vi "Calibrate and Load.vi"(8 "Calibration Cluster":T1, 9 "Always Calibrate":bool, 10 "Do Not Calibrate":bool, 11 "IO Cluster In":T2={"Error"={"status"=FALSE, "code"=0, "source"=""}, "Encoder Calibration Values"=[22, 216], "Update Calibration"=FALSE, "JPEG Resolutions"=3, "Raw Resolutions"=1, "Image Mode"=enum."RAW Gray Scale", "FPGA Ref"=refnum} {"JPEG Resolutions" items=["160x128"=3, "320x240"=5, "640x480"=7]; "Raw Resolutions" items=["80x60"=1, "160x120"=3, "128x128"=9, "128x96"=11]}) -> (0 "Exit Loop":bool, 2 "State Out":T3, 3 "IO Cluster Out":T2={"Error"={"status"=FALSE, "code"=0, "source"=""}, "Encoder Calibration Values"=[22, 216], "Update Calibration"=FALSE, "JPEG Resolutions"=3, "Raw Resolutions"=1, "Image Mode"=enum."RAW Gray Scale", "FPGA Ref"=refnum} {"JPEG Resolutions" items=["160x128"=3, "320x240"=5, "640x480"=7]; "Raw Resolutions" items=["80x60"=1, "160x120"=3, "128x128"=9, "128x96"=11]})   [LabVIEW 2019]
uses:
  Operation States.ctl
  QNET MS IO Cluster.ctl
  <vilib>/Utility/error.llb/Error Cluster From Error Code.vi
  <vilib>/rvi/errors/niLvFpgaAdjustHostInterfaceError.vi
  <vilib>/rvi/interface/nirviReadWriteControl/nirviReadWriteControl.xnode
  NiFpgaLv.dll
  <vilib>/rvi/interface/Simulation/niFpgaSimulationCallBeginRW.vi
panel:
  out "Close Enough?":bool
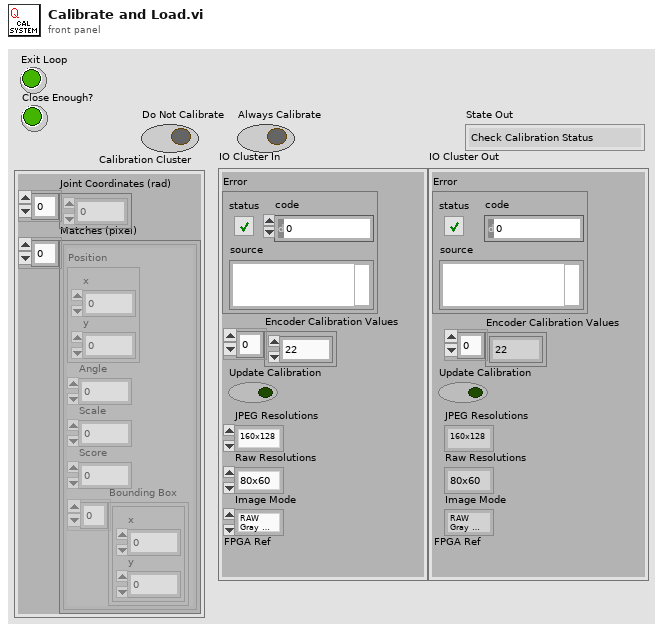
[diagram p1: front panel]
types:
  T1 = cluster{"Joint Coordinates (rad)":dbl[], "Matches (pixel)":cluster{"Position":cluster{"x":sgl, "y":sgl}, "Angle":sgl, "Scale":sgl, "Score":sgl, "Bounding Box":cluster{"x":sgl, "y":sgl}[]}[]}
  T2 = typedef "QNET MS IO Cluster.ctl" = cluster{"Error":errorcluster, "Encoder Calibration Values":i32[], "Update Calibration":bool, "JPEG Resolutions":u16, "Raw Resolutions":u16, "Image Mode":enum16{"RAW RGB", "RAW Gray Scale", "JPEG"}, "FPGA Ref":refnum<k20>}
  T3 = typedef "Operation States.ctl" = enum16{"Check Calibration Status", "Move to Hard Stops", "Calibrate on Symbol", "Calibration Done"}
  T4 = cluster{"Position":cluster{"x":sgl, "y":sgl}, "Angle":sgl, "Scale":sgl, "Score":sgl, "Bounding Box":cluster{"x":sgl, "y":sgl}[]}[]
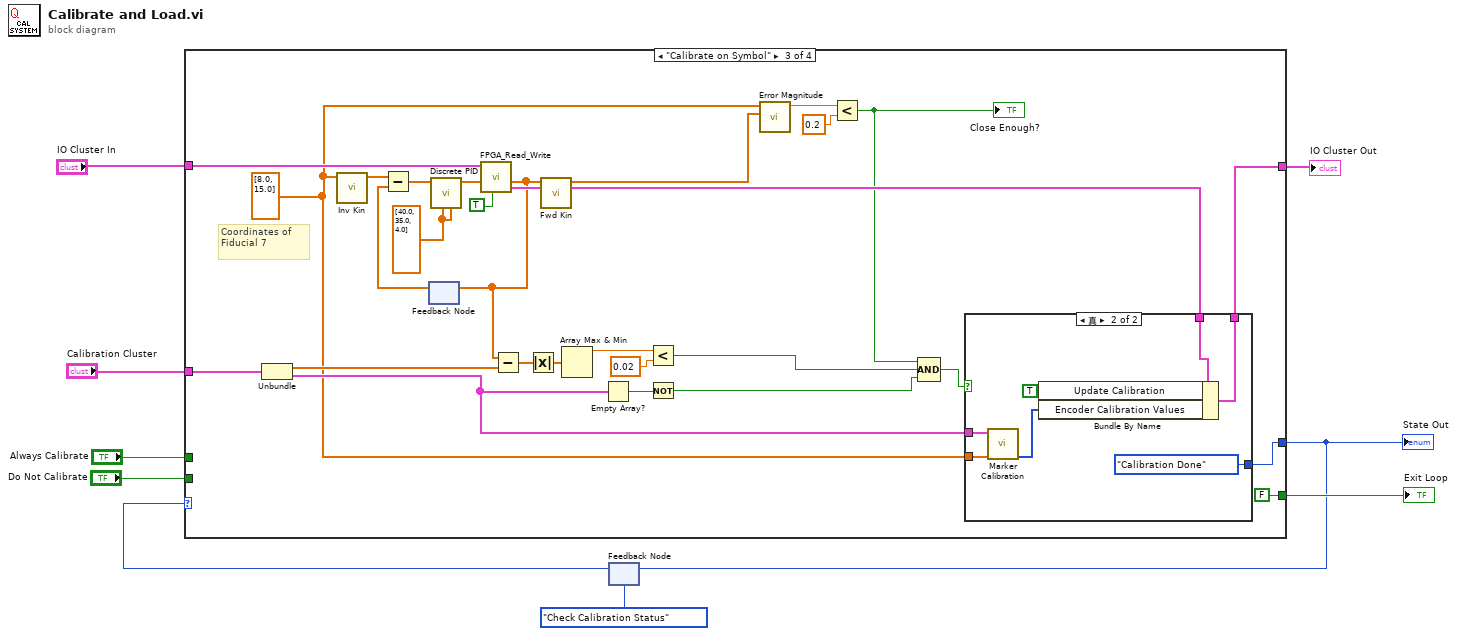
[diagram p0: block diagram]
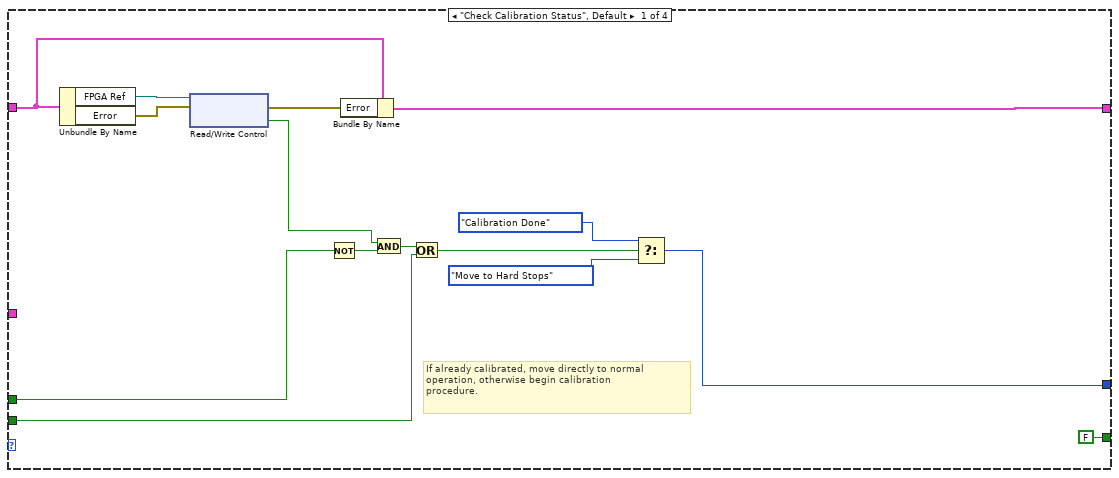
[diagram p2: hidden frame]
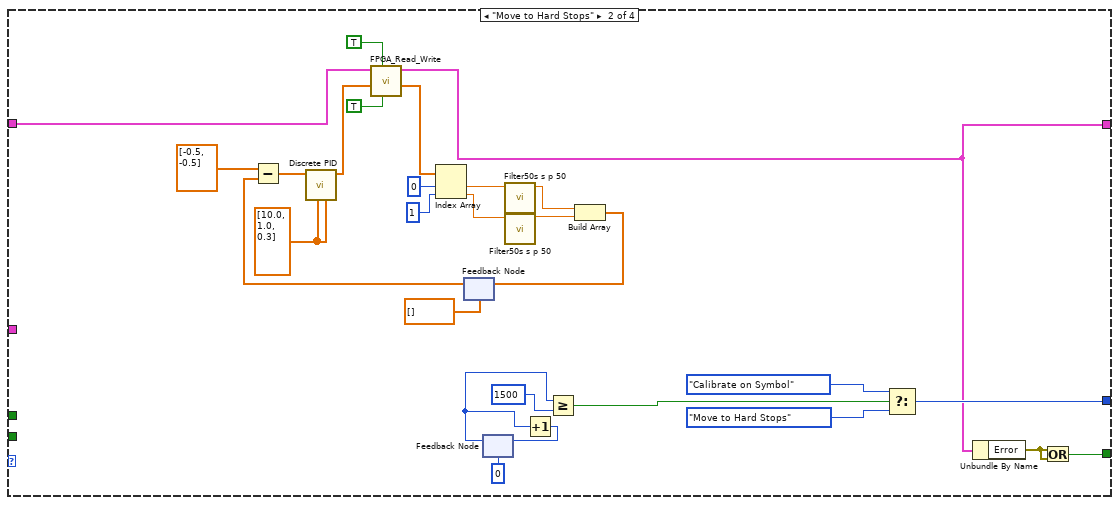
[diagram p3: hidden frame]
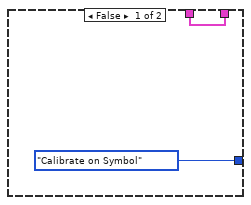
[diagram p4: hidden frame]
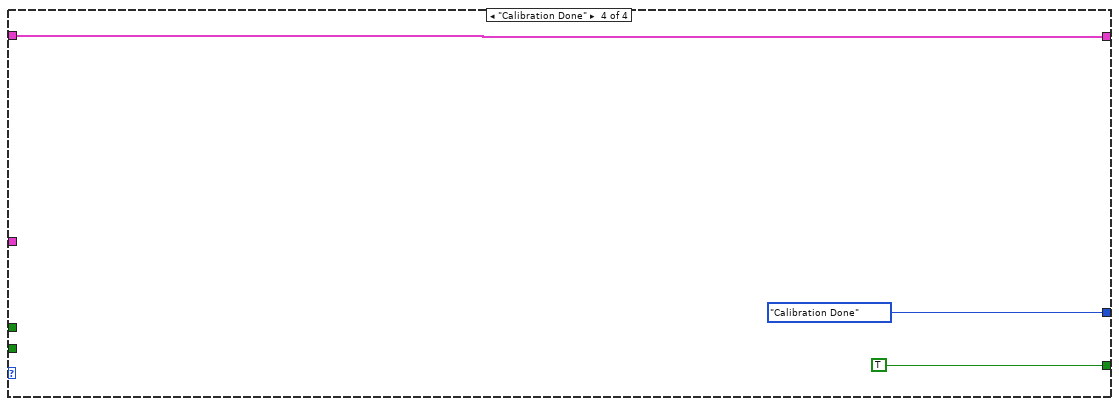
[diagram p5: hidden frame]
diagram:
  n1 = feedback #1(Operation_States."Check Calibration Status") -> (w6:T3)
  n2 = case shown="\"Calibrate on Symbol\"" w6 {
    tunnel: "IO Cluster In" -> [w21 w31 w80 w91]
    tunnel: [FALSE w46 FALSE TRUE] -> w9
    tunnel: [w11 w28 w73 w91] -> w3
    tunnel: [w19 w50 w65 Operation_States."Calibration Done"] -> w5
    tunnel: "Always Calibrate" -> [w16 _ _ _]
    tunnel: "Do Not Calibrate" -> [w13 _ _ _]
    tunnel: "Calibration Cluster" -> [_ _ w68 _]
    frame "Check Calibration Status", Default {
      # "If already calibrated, move directly to normal\noperation, otherwise begin calibration\nprocedure."
      n3 = Unbundle By Name(w21) -> ("FPGA Ref"=w23:refnum<k20>, "Error"=w22:errorcluster)
      n4 = xnode "Read/Write Control"("FPGA VI引用输入"=w23, "错误输入"=w22) -> ("错误输出"=w24:errorcluster, "Calibrated"=w15:bool)  [unwired: 1 out]
      n5 = Not(x=w16) -> (.not. x?=w17:bool)
      n6 = Bundle By Name(cluster=w21, "Error"=w24) -> (w11:T2)
      n7 = And(x=w15, y=w17) -> (x .and. y?=w14:bool)
      n8 = Or(x=w14, y=w13) -> (x .or. y?=w12:bool)
      n9 = Select(t=Operation_States."Calibration Done", s=w12, f=Operation_States."Move to Hard Stops") -> (s? t:f=w19:T3)
    }
    frame "Move to Hard Stops" {
      w35 = dbl[] [10.0, 1.0, 0.3] ("Gains Motor 1")
      n10 = feedback #2(dbl[] []) -> (w38:dbl[])
      n11 = Subtract(x=dbl[] [-0.5, -0.5], y=w38) -> (x-y=w36:dbl[])
      n12 = call "Discrete PID.vi"("Gains Motor 1"=w35, "Gains Motor 0"=w35, "Error Array"=w36) -> ("Voltage"=w25:dbl[])  [unwired: 8 in]
      n13 = call "FPGA_Read_Write.vi"("Motors enabled?"=TRUE, "Reset Encoders?"=TRUE, "Commands"=w25, "IO Cluster In"=w31) -> ("Joint Coordinates (rad)"=w29:dbl[], "IO Cluster Out"=w28:T2)  [unwired: 4 in, 2 out]
      n14 = Index Array(array=w29, index #1=0 ("index"), index #2=1 ("index 2")) -> (element #1=w43:dbl, element #2=w42:dbl)
      n15 = feedback #3(0 ("x")) -> (w32:i32)
      n16 = call "Filter50s s p 50.vi"("u"=w43) -> ("y"=w41:dbl)  [unwired: 10 in]
      n17 = call "Filter50s s p 50.vi"("u"=w42) -> ("y"=w40:dbl)  [unwired: 10 in]
      n18 = Increment(x=w32) -> (x+1=w51:i32)
      n19 = feedback-in #3(w51) -> ()
      n20 = Greater Or Equal?(x=w32, y=1500 ("x")) -> (x >= y?=w27:bool)
      n21 = Build Array(w41, w40) -> (w39:dbl[])
      n22 = feedback-in #2(w39) -> ()
      n23 = Select(t=Operation_States."Calibrate on Symbol" ("f"), s=w27, f=Operation_States."Move to Hard Stops") -> (s? t:f=w50:T3)
      n24 = Unbundle By Name(w28) -> ("Error"=w47:errorcluster)
      n25 = Or(x=w47, y=w47) -> (x .or. y?=w46:bool)
    }
    frame "Calibrate on Symbol" {
      w53 = dbl[] [8.0, 15.0] ("appended array")
      w69 = dbl[] [40.0, 35.0, 4.0] ("appended array")
      # "Coordinates of\nFiducial 7"
      n26 = Unbundle(w68) -> ("Joint Coordinates (rad)"=w62:dbl[], "Matches (pixel)"=w67:T4)
      n27 = call "Inv Kin.vi"("Task Coordinates (cm)"=w53) -> ("Joint Coordinates (rad)"=w75:dbl[])  [unwired: 10 in]
      n28 = feedback #4 ("Feedback Node 2")() -> (w74:dbl[])  [unwired: 1 in]
      n29 = Subtract ("Subtract 3")(x=w75, y=w74) -> (x-y=w76:dbl[])
      n30 = call "Discrete PID.vi"("Gains Motor 1"=w69, "Gains Motor 0"=w69, "Error Array"=w76) -> ("Voltage"=w77:dbl[])  [unwired: 8 in]
      n31 = call "FPGA_Read_Write.vi"("Motors enabled?"=TRUE ("Motors Enabled"), "Commands"=w77, "IO Cluster In"=w80) -> ("Joint Coordinates (rad)"=w63:dbl[], "IO Cluster Out"=w72:T2)  [unwired: 5 in, 2 out]
      n32 = feedback-in #4 ("3")(w63) -> ()
      n33 = Subtract(x=w63, y=w62) -> (x-y=w61:dbl[])
      n34 = Absolute Value(x=w61) -> (abs(x)=w60:dbl[])
      n35 = call "Fwd Kin.vi"("Joint Coordinates (rad)"=w63) -> ("Task Coordinates (cm)"=w71:dbl[])  [unwired: 9 in, 1 out]
      n36 = Array Max & Min(array=w60) -> (max value=w59:dbl)  [unwired: 3 out]
      n37 = Empty Array?(array=w67) -> (empty?=w66:bool)
      n38 = Less?(x=w59, y=0.02) -> (x < y?=w56:bool)
      n39 = Not(x=w66) -> (.not. x?=w55:bool)
      n40 = call "Error Magnitude.vi"("Actual Task Coordinates (cm)"=w71, "Desired Task Coordinates (cm)"=w53) -> ("Task-space\nError"=w70:dbl)  [unwired: 9 in]
      n41 = Less?(x=w70, y=0.2) -> (x < y?=w57:bool)
      "Close Enough?" <- w57
      n42 = Compound Arithmetic op=AND(w57, w56, w55) -> (w54:bool)
      n43 = case shown="真" w54 {
        tunnel: [w81 w89] -> w73
        tunnel: w72 -> [w81 w84]
        tunnel: w67 -> [_ w88]
        tunnel: [Operation_States."Calibrate on Symbol" ("f") Operation_States."Calibration Done" ("t")] -> w65
        tunnel: w53 -> [_ w83]
        frame False {
        }
        frame True {
          n44 = call "Marker Calibration.vi"("Marker Location"=w83, "Match"=w88) -> ("Encoder Setpoint"=w86:i32[])  [unwired: 7 in, 2 out]
          n45 = Bundle By Name(cluster=w84, "Update Calibration"=TRUE, "Encoder Calibration Values"=w86) -> (w89:T2)
        }
      }
    }
    frame "Calibration Done" {
    }
  }
  "State Out" <- w5
  "Exit Loop" <- w9
  "IO Cluster Out" <- w3
  n46 = feedback-in #1(w5) -> ()
